vi "read_radius.vi"(8 "error in (no error)":errorcluster, 11 "RNeighbors in":refnum<class "RNeighbors.lvclass">) -> (0 "error out":errorcluster, 2 "radius":dbl=1.0, 3 "RNeighbors out":refnum<class "RNeighbors.lvclass">)   [LabVIEW 2020, in "RNeighbors.lvclass"]
uses:
  RNeighbors.lvclass
  RNeighbors.lvclass/RNeighbors.ctl
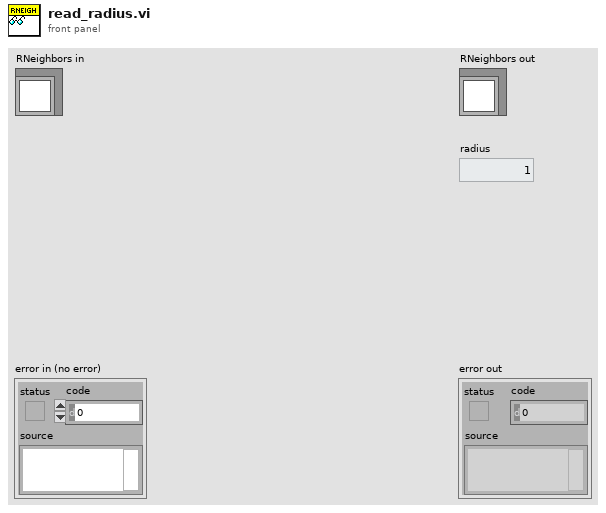
[diagram p1: front panel]
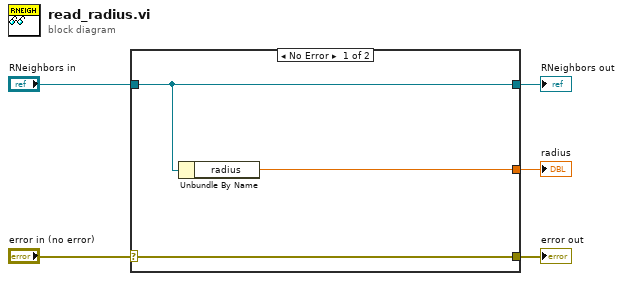
[diagram p0: block diagram]
diagram:
  n1 = case shown="No Error" "error in (no error)" {
    selector: "error in (no error)" -> [w8 w9]
    tunnel: [w8 w9] -> w4
    tunnel: [w7 w10] -> w2
    tunnel: "RNeighbors in" -> [w7 w10]
    tunnel: [w6 _] -> w1
    frame No Error {
      n2 = Unbundle By Name(w7) -> ("radius"=w6:dbl)
    }
    frame Error {
    }
  }
  "error out" <- w4
  "RNeighbors out" <- w2
  "radius" <- w1
